vi "Tree_Get Disabled Elements.vi"(8 "error in (no error)":errorcluster, 11 "TreeControl in":refnum<vi>) -> (0 "error out":errorcluster, 1 "Disabled Item Tags":string[](array[string]), 2 "Disabled Elements":bool[](array[boolean]), 3 "TreeControl out":refnum<vi>, 4 "Enabled Item Tags":string[](array[string]))   [LabVIEW 2023]
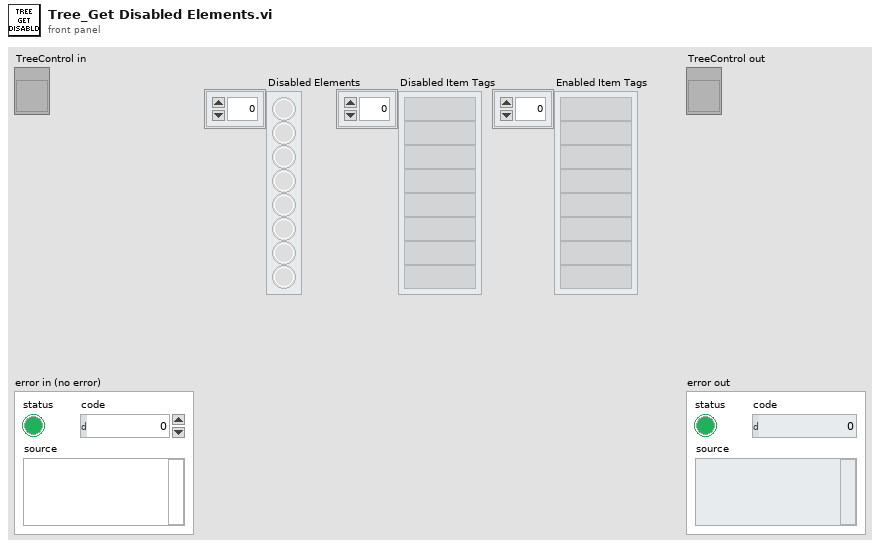
[diagram p1: front panel]
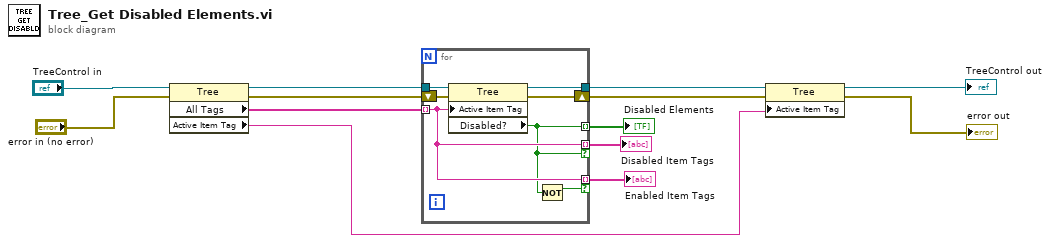
[diagram p0: block diagram]
diagram:
  n1 = property class="Tree"(reference="TreeControl in", error in="error in (no error)") -> (reference out=w10:refnum<vi>, error out=w6:errorcluster, "All Tags"=w12:string[], "Active Item Tag"=w7:string)
  n2 = for {
    tunnel: w10 -> [w20]
    tunnel: w12 -> [w16] mode=indexing
    tunnel: [w15] -> w13 mode=indexing
    tunnel: [w19] -> w9
    shift-right: [w17] -> w5
    shift-left: w6 -> [w18]
    tunnel: [w16] -> w2 mode=indexing if=w15
    tunnel: [w16] -> w1 mode=indexing if=w14
    n3 = property class="Tree"(reference=w20, error in=w18, "Active Item Tag"=w16) -> (reference out=w19:refnum<vi>, error out=w17:errorcluster, "Disabled?"=w15:bool)
    n4 = Not(x=w15) -> (.not. x?=w14:bool)
  }
  "Disabled Elements" <- w13
  "Disabled Item Tags" <- w2
  "Enabled Item Tags" <- w1
  n5 = property on="Property Node" class="Tree"(reference=w9, error in=w5, "Active Item Tag"=w7) -> (reference out=→"TreeControl out":refnum<vi>, error out=→"error out":errorcluster)
